vi "Keithley 6517A LTCC Single Read with Zero Check .vi"(8 "error in":T1, 9 "Read Displays":bool=TRUE, 10 "Scanner Channel":i16=1 min=1 max=10 step=1, 11 "GPIB address":string="1:27") -> (0 "error out":T1, 1 "time and date stamp":string="03:56:06.00,15-Jul-  94", 2 "Time":string="03:56:06.00", 3 "measurement":dbl=-0.063534 format="%.6e", 4 "secondary display":string="\"               Vsource:+000.000V\"\n", 5 "units":string="VDC", 6 "reading #":dbl=1512.0, 7 "primary display":string="\"-0.063534 V CH01    \"\n")   [LabVIEW 2013]
doc: "This VI takes a single reading from the 6517. The data returned includes the reading, timestamp, units, and reading#."
panel:
  in  "Zero Check":bool=TRUE
  out "Raw Readback":string="-0.063534E+00VDC,03:56:06.00,15-Jul-  94,+01512RDNG#\n"
  # "(A)"
  # "ON\nOFF"
  # "ON\nOFF"
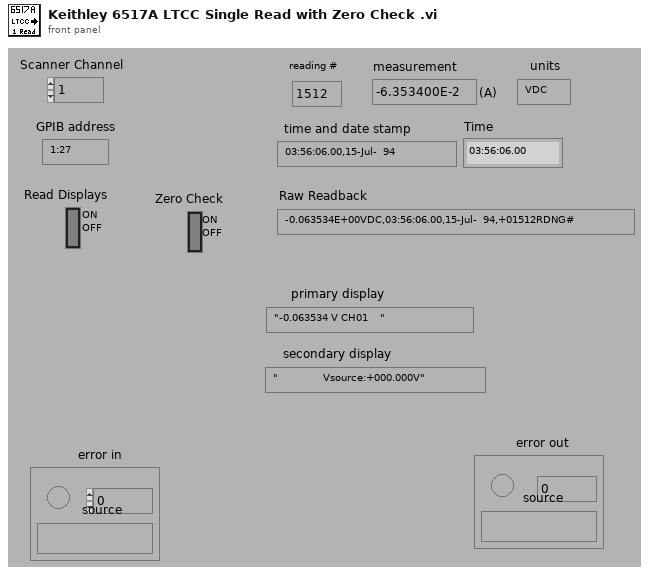
[diagram p1: front panel]
types:
  T1 = cluster{"error":bool, "code":i32, "source":string}
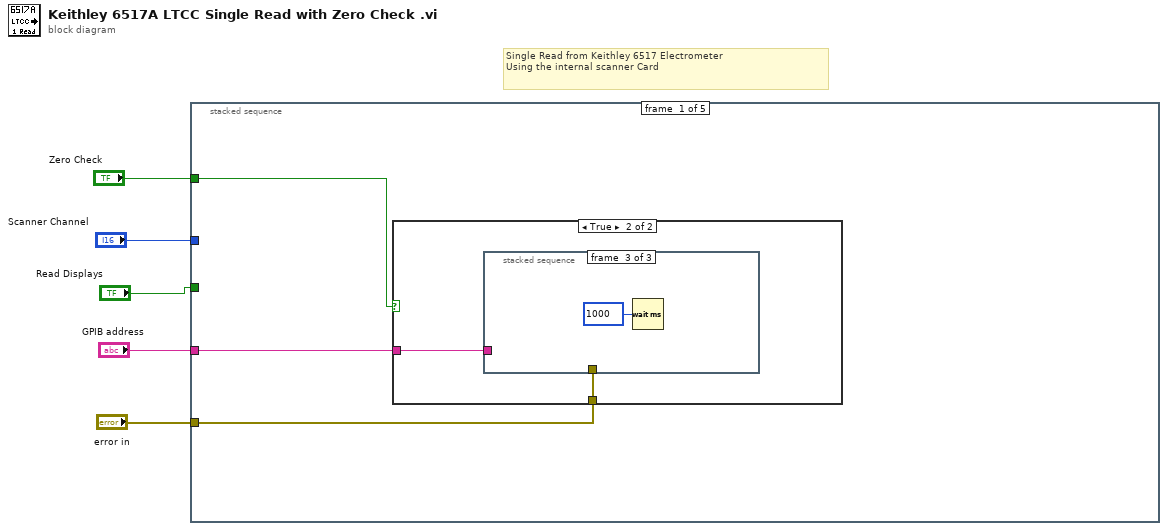
[diagram p0: block diagram]
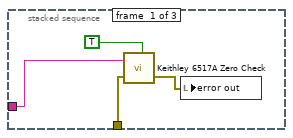
[diagram p3: hidden frame]
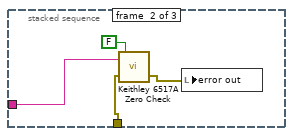
[diagram p4: hidden frame]
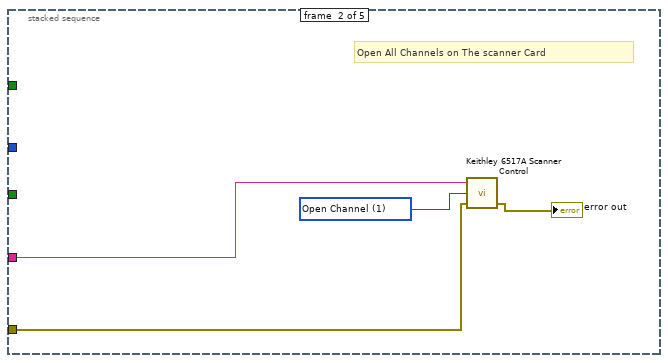
[diagram p5: hidden frame]
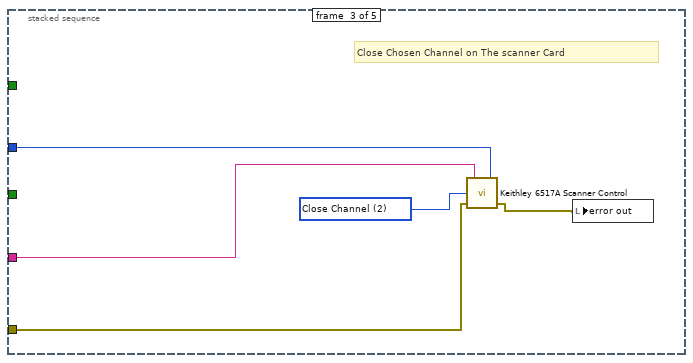
[diagram p6: hidden frame]
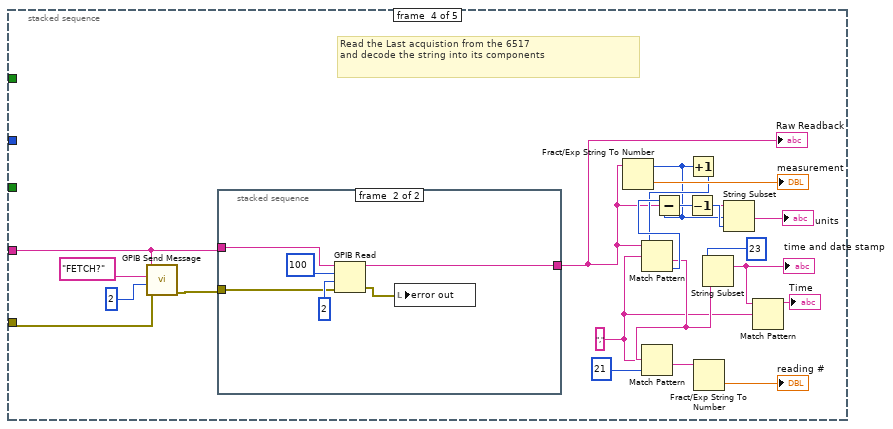
[diagram p7: hidden frame]
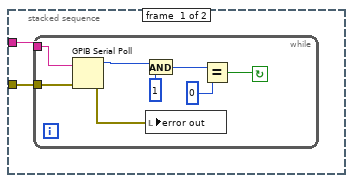
[diagram p8: hidden frame]
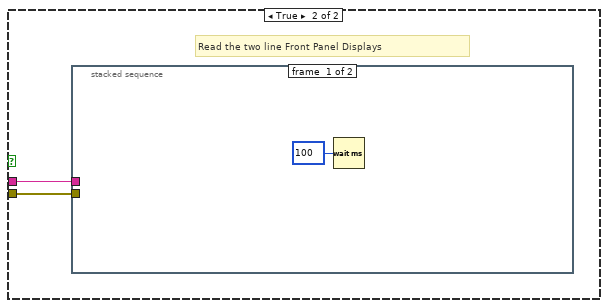
[diagram p10: hidden frame]
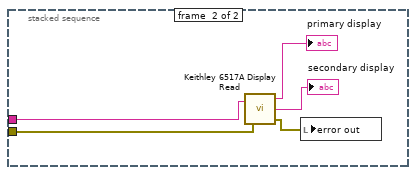
[diagram p11: hidden frame]
diagram:
  # "Single Read from Keithley 6517 Electrometer \nUsing the internal scanner Card"
  n1 = stacked-sequence {
    tunnel: "GPIB address" -> [w6 w20 w26 w34 w67]
    tunnel: "error in" -> [w7 w23 w28 w32 w66]
    tunnel: "Scanner Channel" -> [_ _ w24 _ _]
    tunnel: "Read Displays" -> [_ _ _ _ w68]
    tunnel: "Zero Check" -> [w8 _ _ _ _]
    frame #0 {
      n2 = case shown="True" w8 {
        tunnel: w7 -> [_ w10]
        tunnel: w6 -> [_ w9]
        frame False {
        }
        frame True {
          n3 = stacked-sequence {
            tunnel: w10 -> [w14 w18 _]
            tunnel: w9 -> [w13 w17 _]
            frame #0 {
              n4 = call "Keithley 6517A Zero Check.vi"("Zero Check"=TRUE, "error in"=w14, "GPIB address"=w13) -> ("error out"=w11:T1)
              n5 = local write "error out"(w11) -> ()
            }
            frame #1 {
              n6 = call "Keithley 6517A Zero Check.vi"("Zero Check"=FALSE, "error in"=w18, "GPIB address"=w17) -> ("error out"=w15:T1)
              n7 = local write "error out"(w15) -> ()
            }
            frame #2 {
              n8 = Wait (ms)(milliseconds to wait=u32 1000) -> ()  [unwired: 1 out]
            }
          }
        }
      }
    }
    frame #1 {
      w22 = u16 1 items=["Open All", "Open Channel", "Close Channel", "Scan List"] ("Scanner Control")
      # "Open All Channels on The scanner Card"
      n9 = call "Keithley 6517A Scanner Control.vi"("error in"=w23, "Scanner Control"=w22, "GPIB address"=w20) -> ("error out"=→"error out":T1)  [unwired: 2 in]
    }
    frame #2 {
      w27 = u16 2 items=["Open All", "Open Channel", "Close Channel", "Scan List"] ("Scanner Control")
      # "Close Chosen Channel on The scanner Card"
      n10 = call "Keithley 6517A Scanner Control.vi"("Open / Close Internal Scanner Channel"=w24, "error in"=w28, "Scanner Control"=w27, "GPIB address"=w26) -> ("error out"=w25:T1)  [unwired: 1 in]
      n11 = local write "error out"(w25) -> ()
    }
    frame #3 {
      w31 = ","
      # "Read the Last acquistion from the 6517\nand decode the string into its components"
      n12 = call "GPIB Send Message.vi"("address string"=w34, "write buffer"="FETCH?", "write mode (set END:0)"=2, "error in"=w32) -> ("error out"=w35:T1)  [unwired: 3 in, 2 out]
      n13 = stacked-sequence {
        tunnel: [_ w65] -> w33
        tunnel: w35 -> [w50 w62]
        tunnel: w34 -> [w51 w61]
        frame #0 {
          n14 = while {
            tunnel: w51 -> [w54]
            tunnel: w50 -> [w53]
            stop <- w58 continue-if-true
            n15 = GPIB Serial Poll(0:w54, 1:w53) -> (2:w57:i16, 4:w52:errorcluster)  [unwired: 1 out]
            n16 = And(x=w57, y=1) -> (x .and. y?=w55:i32)
            n17 = local write "error out"(w52) -> ()
            n18 = Equal?(x=w55, y=0) -> (x = y?=w58:bool)
          }
        }
        frame #1 {
          n19 = GPIB Read(0:w61, 1:100, 2:2, 3:w62) -> (5:w65:string, 7:w60:errorcluster)  [unwired: 1 in, 1 out]
          n20 = local write "error out"(w60) -> ()
        }
      }
      "Raw Readback" <- w33
      n21 = Fract/Exp String To Number(string=w33) -> (offset past number=w38:i32, number=→"measurement":dbl)  [unwired: 3 in]
      n22 = Increment(x=w38) -> (x+1=w39:i32)
      n23 = Match Pattern(string=w33, regular expression=w31, offset (0)=w39) -> (after substring=w41:string, offset past match=w45:i32)  [unwired: 2 out]
      n24 = Match Pattern(string=w41, regular expression=w31, offset (0)=21) -> (after substring=w46:string)  [unwired: 3 out]
      n25 = Subtract(x=w45, y=w38) -> (x-y=w43:i32)
      n26 = Decrement(x=w43) -> (x-1=w44:i32)
      n27 = Fract/Exp String To Number(string=w46) -> (number=→"reading #":dbl)  [unwired: 3 in, 1 out]
      n28 = String Subset(string=w41, length (rest)=23) -> (substring=w30:string)  [unwired: 1 in]
      "time and date stamp" <- w30
      n29 = String Subset(string=w33, offset (0)=w38, length (rest)=w44) -> (substring=→"units":string)
      n30 = Match Pattern(string=w30, regular expression=w31) -> (before substring=→"Time":string)  [unwired: 1 in, 3 out]
    }
    frame #4 {
      n31 = case shown="False" w68 {
        tunnel: w67 -> [_ w70]
        tunnel: w66 -> [_ w69]
        frame False {
        }
        frame True {
          # "Read the two line Front Panel Displays"
          n32 = stacked-sequence {
            tunnel: w70 -> [_ w76]
            tunnel: w69 -> [_ w75]
            frame #0 {
              n33 = Wait (ms)(milliseconds to wait=u32 100) -> ()  [unwired: 1 out]
            }
            frame #1 {
              n34 = call "Keithley 6517A Display Read.vi"("GPIB address"=w76, "error in"=w75) -> ("primary display"=→"primary display":string, "secondary display"=→"secondary display":string, "error out"=w72:T1)
              n35 = local write "error out"(w72) -> ()
            }
          }
        }
      }
    }
  }
